vi "Tusk.KillAll(Local).vi"(8 "error in (no error)":errorcluster, 9 "Data":variant, 11 "Tusk in":refnum<class "Tusk.lvclass">) -> (0 "error out":errorcluster, 3 "Tusk out":refnum<class "Tusk.lvclass">)   [LabVIEW 2018, in "Application.lvlib" / "Tusk.lvclass"]
uses:
  Tusk.lvclass
  Tusk.lvclass/Tusk.ctl
  Message Class/Message.lvclass/Message.ctl
  Dictionary Class/Dictionary.lvclass/Dictionary.ctl
  Tusk.GetDictionary.vi
  Tusk.MessageAllSenderCore.vi/1679c56e-e765-44f0-aff8-f47c4dbf3d60.vi
  Tusk.MessageSenderCore.vi
  Dictionary Class/VIs/Get Data DVR.vi
  Exceptions Class/VIs/Invalid Type.vi
  <vilib>/Utility/error.llb/Trim Whitespace.vi
  Message Class/Message.lvclass
  Keywords Class/Keywords.lvclass
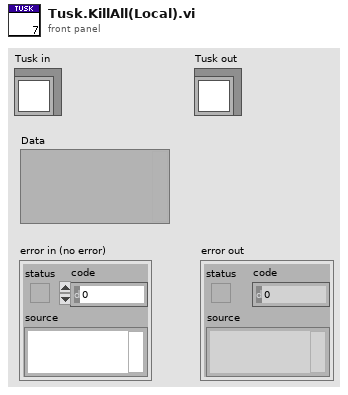
[diagram p1: front panel]
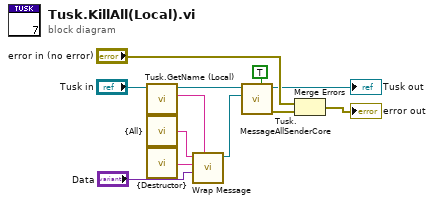
[diagram p0: block diagram]
diagram:
  n1 = call "Tusk.GetName (Local).vi"("Tusk in"="Tusk in") -> ("Name(Local)"=w10:string, "Tusk out"=w5:refnum<class "Tusk.lvclass">)  [unwired: 8 in, 1 out]
  n2 = call "{All}.vi"() -> ("Word"=w1:string)  [unwired: 6 in]
  n3 = call "{Destructor}.vi"() -> ("Word"=w9:string)  [unwired: 6 in]
  n4 = call "Wrap Message.vi"("Sender"=w10, "Data"="Data", "Message"=w9, "Recipient"=w1) -> ("Message out"=w2:refnum<class "Message.lvclass">)  [unwired: 6 in, 1 out]
  n5 = call "Tusk.MessageAllSenderCore.vi"("Priority?"=TRUE, "Message"=w2, "Tusk in"=w5) -> ("error out"=w6:errorcluster, "Tusk out"=→"Tusk out":refnum<class "Tusk.lvclass">)  [unwired: 7 in]
  n6 = Merge Errors("error in (no error)", w6) -> (→"error out":errorcluster)
